vi "Add Node (Extended).vi"(8 "error in (no error)":errorcluster, 9 "Assertions":T1[](array[typedef]), 10 "Test Node":T2, 11 "Test Result in":refnum<class "Test Result.lvclass">) -> (0 "error out":errorcluster, 3 "Test Result out":refnum<class "Test Result.lvclass">)   [LabVIEW 2020, in "Caraya.lvlib" / "Test Result.lvclass"]
uses:
  Test Result.lvclass
  Test Node (Extended).ctl
  Test Registration Data.ctl
  Assert Event Data (Extended).ctl
  Test Result.lvclass/Test Result.ctl
  Caraya.lvlib
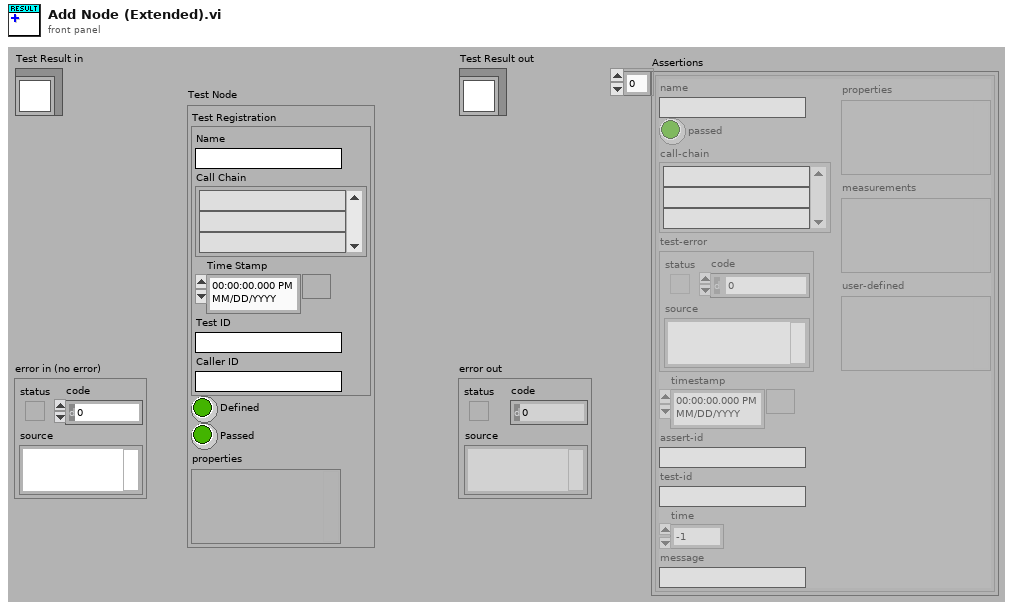
[diagram p1: front panel]
types:
  T1 = typedef "Caraya.lvlib/Test Result.lvclass/Assert Event Data (Extended).ctl" = cluster{"name":string, "passed":bool, "call-chain":string[], "test-error":errorcluster, "timestamp":timestamp, "assert-id":string, "test-id":string, "time":dbl, "message":string, "properties":variant, "measurements":variant, "user-defined":variant}
  T2 = typedef "Caraya.lvlib/Test Result.lvclass/Test Node (Extended).ctl" = cluster{"Test Registration":T3, "Defined":bool, "Passed":bool, "properties":variant}
  T3 = typedef "Caraya.lvlib/Test Result.lvclass/Test Registration Data.ctl" = cluster{"Name":string, "Call Chain":string[], "Time Stamp":timestamp, "Test ID":string, "Caller ID":string}
  T4 = typedef "Caraya.lvlib/Test Result.lvclass/Node Results (Extended).ctl" = cluster{"Test Node":T2, "Assertions":T1[]}
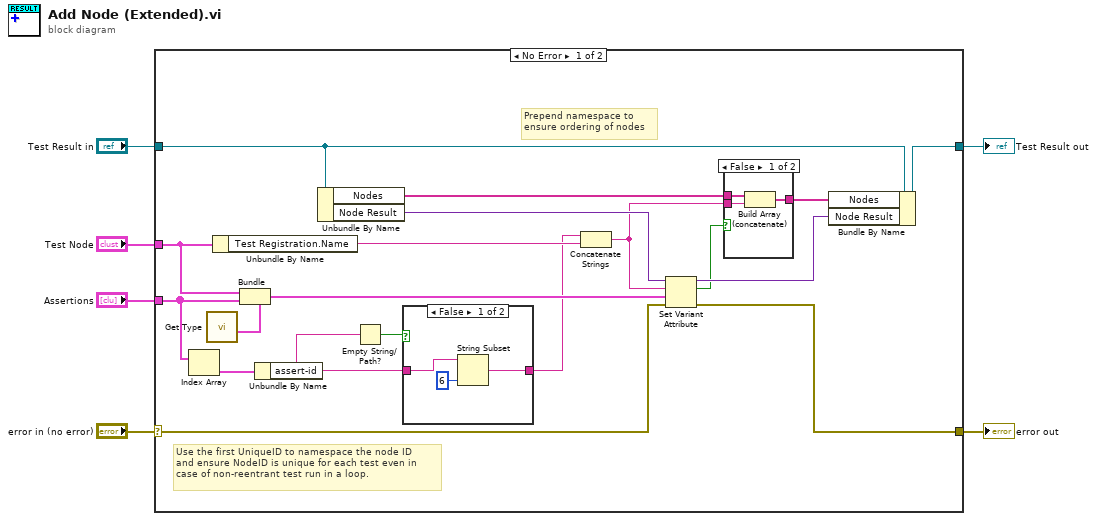
[diagram p0: block diagram]
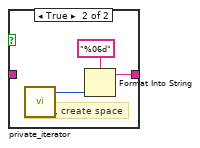
[diagram p3: hidden frame]
diagram:
  n1 = case shown="No Error" "error in (no error)" {
    selector: "error in (no error)" -> [w17 w37]
    tunnel: [w16 w37] -> w5
    tunnel: [w24 w36] -> w3
    tunnel: "Test Result in" -> [w25 w36]
    tunnel: "Test Node" -> [w21 _]
    tunnel: "Assertions" -> [w13 _]
    frame No Error {
      # "Prepend namespace to\nensure ordering of nodes"
      # "Use the first UniqueID to namespace the node ID\nand ensure NodeID is unique for each test even in \ncase of non-reentrant test run in a loop."
      n2 = Index Array(array=w13) -> (element=w12:T1)  [unwired: 1 in]
      n3 = call "Get Type.vi"() -> ("Extended Node Result"=w8:T4)  [unwired: 10 in, 1 out]
      n4 = Unbundle By Name(w21) -> ("Test Registration.Name"=w15:string)
      n5 = Bundle(cluster=w8, "Test Node"=w21, "Assertions"=w13) -> (w19:T4)
      n6 = Unbundle By Name(w12) -> ("assert-id"=w10:string)
      n7 = Unbundle By Name(w25) -> ("Nodes"=w23:string[], "Node Result"=w20:variant)
      n8 = Empty String/Path?(string/path=w10) -> (empty?=w11:bool)
      n9 = case shown="False" w11 {
        tunnel: w10 -> [w31 _]
        tunnel: [w30 w35] -> w9
        frame False {
          n10 = String Subset(string=w31, length (rest)=6 ("length (rest)")) -> (substring=w30:string)  [unwired: 1 in]
        }
        frame True {
          # "If test, create space"
          n11 = call "private_iterator.vi"() -> ("iterator"=w34:u32)  [unwired: 11 in]
          n12 = Format Into String(format string="%06d", w34) -> (resulting string=w35:string)  [unwired: 2 in, 1 out]
        }
      }
      n13 = Concatenate Strings(w9, w15) -> (w14:string)
      n14 = Set Variant Attribute(Variant=w20, name=w14, value=w19, error in=w17) -> (Variant out=w18:variant, replaced=w7:bool, error out=w16:errorcluster)
      n15 = case shown="False" w7 {
        tunnel: w23 -> [w28 w29]
        tunnel: [w27 w29] -> w22
        tunnel: w14 -> [w26 _]
        frame False {
          n16 = Build Array (concatenate)(w28, w26) -> (w27:string[])
        }
        frame True {
        }
      }
      n17 = Bundle By Name(cluster=w25, "Nodes"=w22, "Node Result"=w18) -> (w24:refnum<class "Test Result.lvclass">)
    }
    frame Error {
    }
  }
  "error out" <- w5
  "Test Result out" <- w3
